vi "Conv_AngleDegrees_Heading.vi"(10 "Degrees":dbl) -> (2 "Heading Degrees":dbl)   [LabVIEW 2019, in "Trajectory_Library.lvlib"]
doc: "Convert angle (degrees) to heading (+/- 180) (degrees)\nNOTE: increases counter clockwise"
uses:
  Trajectory_Library.lvlib
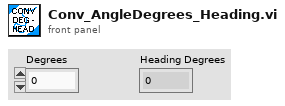
[diagram p1: front panel]
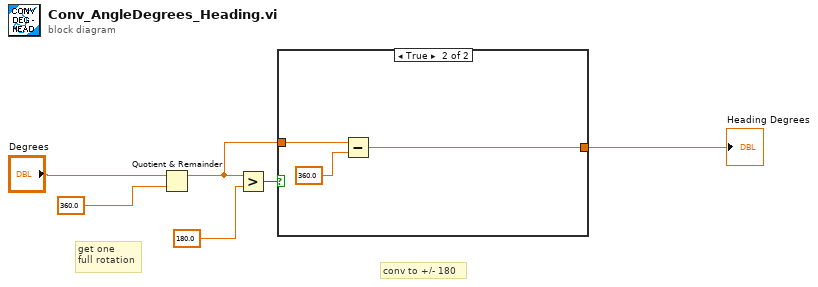
[diagram p0: block diagram]
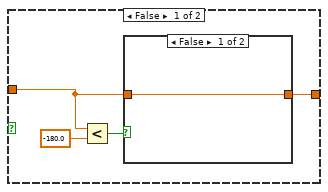
[diagram p2: hidden frame]
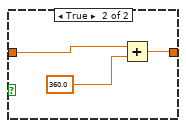
[diagram p3: hidden frame]
diagram:
  # "get one\nfull rotation"
  # "conv to +/- 180"
  n1 = Quotient & Remainder(x="Degrees", y=360.0) -> (x-y*floor(x/y)=w2:dbl)  [unwired: 1 out]
  n2 = Greater?(x=w2, y=180.0) -> (0:w3:bool)
  n3 = case shown="True" w3 {
    tunnel: w2 -> [w9 w16]
    tunnel: [w8 w15] -> w1
    frame False {
      n4 = Less?(x=w9, y=-180.0) -> (x < y?=w10:bool)
      n5 = case shown="False" w10 {
        tunnel: w9 -> [w11 w13]
        tunnel: [w11 w14] -> w8
        frame False {
        }
        frame True {
          n6 = Add(x=w13, y=360.0) -> (x+y=w14:dbl)
        }
      }
    }
    frame True {
      n7 = Subtract(x=w16, y=360.0) -> (x-y=w15:dbl)
    }
  }
  "Heading Degrees" <- w1
